vi "SAVE_FILE_DIALOG.vi"(0 "Enable":bool=TRUE, 5 "error in (no error)":errorcluster) -> (12 "Cancel 2":bool, 14 "FREQUENCY 2":string(combo), 15 "SUM/DELTA 2":string(combo), 16 "POLARIZATION 2":string(combo), 17 "Diagnostics 3":string, 18 "OK":bool, 19 "error out":errorcluster)   [LabVIEW 2017]
doc: "Displays a standard dialog box that prompts users to enter information, such as a user name and password."
panel:
  in  "DIAGNOSTICS":string
  in  "FREQUENCY":string(combo)="5400"
  in  "SUM/DELTA":string(combo)="DELTA"
  in  "POLARIZATION":string(combo)="AZ"
  out "String":string
  in  "Cancel":bool
  in  "OK2":bool
  in  "OK1":bool
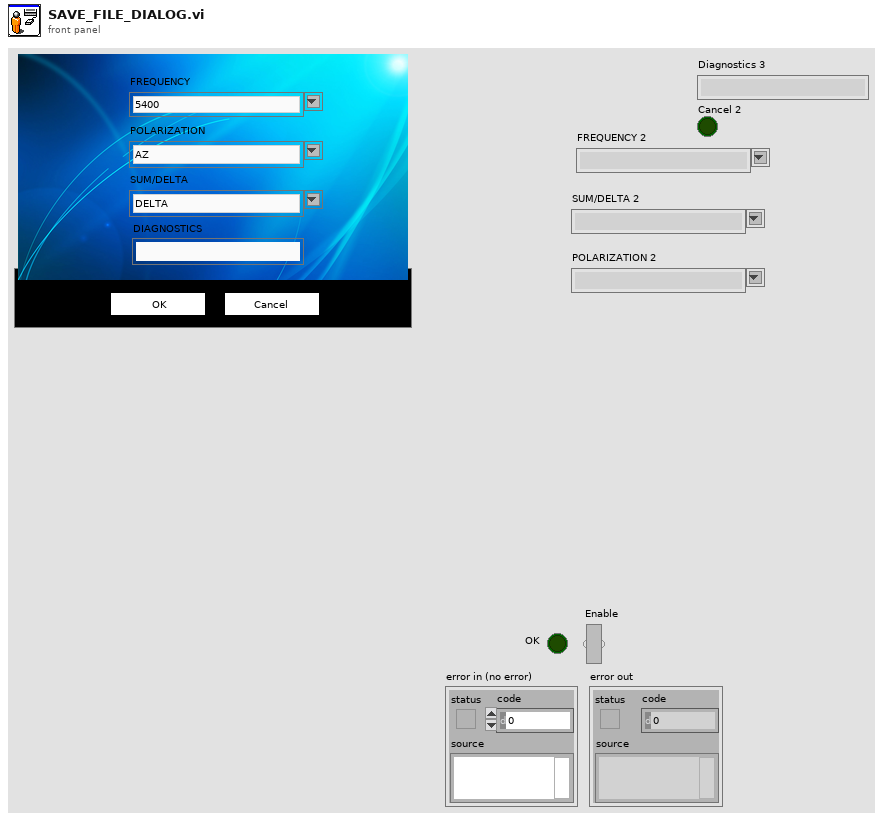
[diagram p1: front panel]
types:
  T1 = cluster{"Input Name":string, "Input Data Type":i32}[]
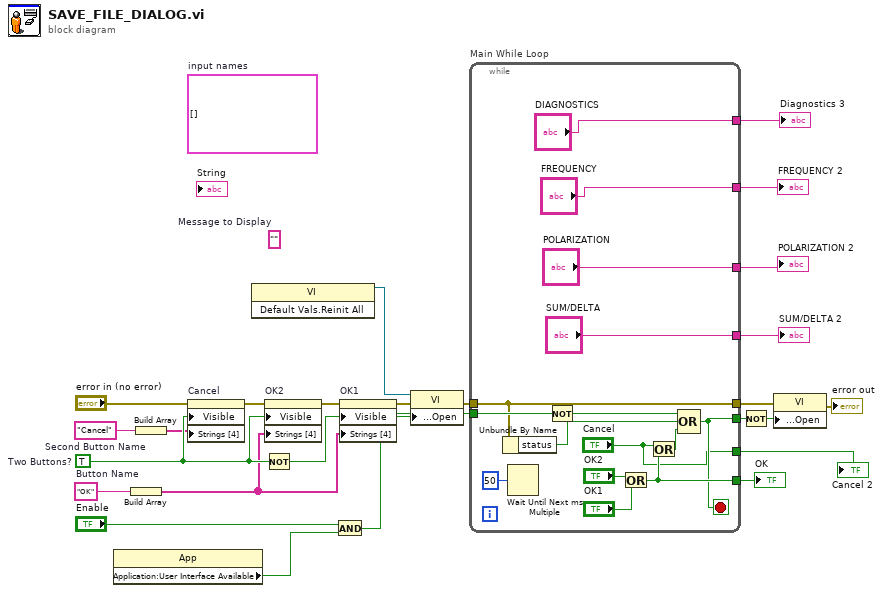
[diagram p0: block diagram]
diagram:
  (unwired) T1 []  # input names
  w17 = "Cancel"  # Second Button Name
  w15 = "OK"  # Button Name
  (unwired) ""  # Message to Display
  w25 = TRUE  # Two Buttons?
  n1 = property class="App"() -> ("Application:User Interface Available"=w7:bool)  [unwired: 2 in, 2 out]
  n2 = Build Array(w15) -> (w16:string[])
  n3 = Build Array(w17) -> (w18:string[])
  n4 = property on="Cancel" class="Bool"(error in="error in (no error)", "Visible"=w25, "Strings [4]"=w18) -> (error out=w22:errorcluster)  [unwired: 1 in, 1 out]
  n5 = invoke class="VI" method="Default Vals.Reinit All"() -> (reference out=w6:refnum<vi>)  [unwired: 3 in, 2 out]
  n6 = Not(x=w25) -> (.not. x?=w23:bool)
  n7 = property on="OK2" class="Bool"(error in=w22, "Visible"=w25, "Strings [4]"=w16) -> (error out=w21:errorcluster)  [unwired: 1 in, 1 out]
  n8 = And(x="Enable", y=w7) -> (x .and. y?=w8:bool)
  n9 = property on="OK1" class="Bool"(error in=w21, "Visible"=w23, "Strings [4]"=w16) -> (error out=w14:errorcluster)  [unwired: 1 in, 1 out]
  n10 = property class="VI"(reference=w6, error in=w14, "Front Panel Window:Open"=w8) -> (error out=w13:errorcluster)  [unwired: 1 out]
  n11 = while "Main While Loop" {
    tunnel: [w38] -> w24
    tunnel: w8 -> [w36]
    tunnel: [w34] -> w19
    tunnel: w13 -> [w33]
    tunnel: [w33] -> w11
    tunnel: ["FREQUENCY"] -> w5
    tunnel: ["POLARIZATION"] -> w4
    tunnel: ["SUM/DELTA"] -> w3
    tunnel: ["DIAGNOSTICS"] -> w2
    tunnel: ["Cancel"] -> w1
    stop <- w34 stop-if-true
    n12 = Unbundle By Name(w33) -> ("status"=w31:bool)
    n13 = Wait Until Next ms Multiple(millisecond multiple=u32 50) -> ()  [unwired: 1 out]
    n14 = Not(x=w36) -> (.not. x?=w35:bool)
    n15 = Or(x="OK2", y="OK1") -> (x .or. y?=w38:bool)
    n16 = Or(x="Cancel", y=w38) -> (x .or. y?=w32:bool)
    n17 = Compound Arithmetic op=OR(w35, w31, w32) -> (w34:bool)
  }
  "OK" <- w24
  "FREQUENCY 2" <- w5
  "POLARIZATION 2" <- w4
  "SUM/DELTA 2" <- w3
  "Diagnostics 3" <- w2
  "Cancel 2" <- w1
  n18 = Not(x=w19) -> (.not. x?=w20:bool)
  n19 = property class="VI"(error in=w11, "Front Panel Window:Open"=w20) -> (error out=→"error out":errorcluster)  [unwired: 1 in, 1 out]
